vi "getLevelFromIndex.vi"(10 "Index":string) -> (1 "Level":string, 2 "Index out":string)   [LabVIEW 2018]
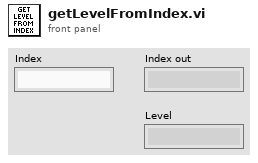
[diagram p1: front panel]
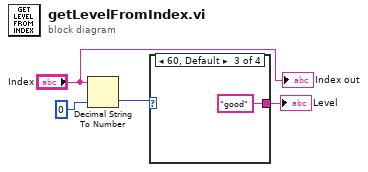
[diagram p0: block diagram]
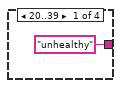
[diagram p2: hidden frame]
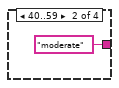
[diagram p3: hidden frame]
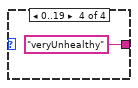
[diagram p4: hidden frame]
diagram:
  n1 = Decimal String To Number(string="Index", default (0L)=u8 0) -> (number=w3:u8)  [unwired: 1 in, 1 out]
  n2 = case shown="60, Default" w3 {
    tunnel: ["unhealthy" "moderate" "good" "veryUnhealthy"] -> w4
    frame 20..39 {
    }
    frame 40..59 {
    }
    frame 60, Default {
    }
    frame 0..19 {
    }
  }
  "Level" <- w4
  "Index out" <- "Index"
